vi "Main.vi"() -> (3 "Script out":refnum<class "Script.lvclass">)   [LabVIEW 2021, in "_Rename.lvlib" / "Script.lvlib" / "Script.lvclass"]
uses:
  Script.lvclass
  Script.lvclass/Script.ctl
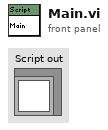
[diagram p1: front panel]
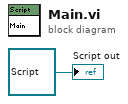
[diagram p0: block diagram]
diagram:
  "Script out" <- refnum<class "Script.lvclass"> refnum ("Script out")
